vi "Large File - Total Measured Energy.vi"(4 "error in":errorcluster, 7 "tdms file":refnum<k34>) -> (0 "error out":errorcluster, 2 "Total Test Energies (J)":dbl[](array[numeric]), 3 "tdms file out":refnum<k34>)   [LabVIEW 2015]
doc: "Calculates the Total Energy of each shot using Trapezoidal Numeric Integration of the Voltage and Current data. This version deals with the large log files by only reading 100,000 data points from the TDMS file at a time for processing."
uses:
  <vilib>/Analysis/8numeric.llb/1D Numeric Integration.vi
  <vilib>/Analysis/NI_AALPro.lvlib
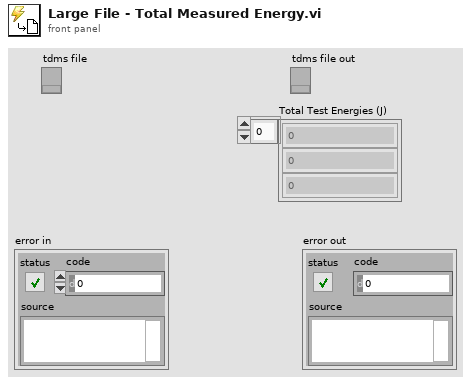
[diagram p1: front panel]
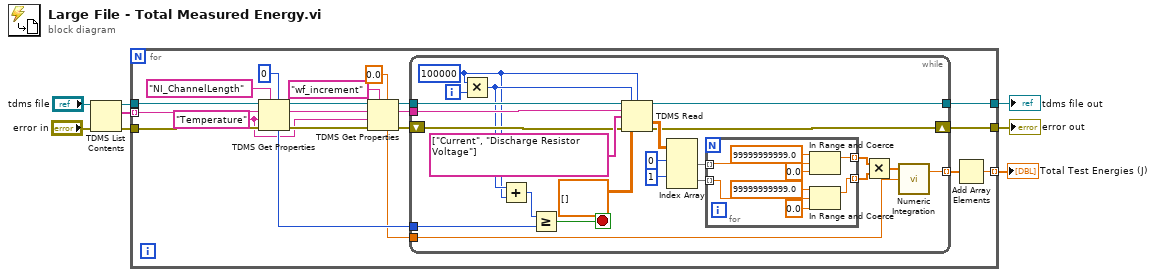
[diagram p0: block diagram]
diagram:
  n1 = TDMS List Contents(4:"error in", 7:"tdms file") -> (0:w7:errorcluster, 2:w6:string[], 3:w8:refnum<k34>)  [unwired: 1 in, 1 out]
  n2 = for {
    tunnel: w8 -> [w22]
    tunnel: [w28] -> w1
    tunnel: w7 -> [w21]
    tunnel: [w27] -> w2
    tunnel: w6 -> [w20] mode=indexing
    tunnel: [w25] -> w5 mode=indexing
    w13 = "Temperature" ("channel name")
    n3 = TDMS Get Properties(5:0, 7:"NI_ChannelLength" ("property name"), 8:w21, 9:w13, 10:w20, 11:w22) -> (0:w18:errorcluster, 2:w16:string, 3:w17:refnum<k34>, 4:w19:i32)  [unwired: 2 out]
    n4 = TDMS Get Properties(5:0.0, 7:"wf_increment" ("property name"), 8:w18, 9:w13, 10:w16, 11:w17) -> (0:w14:errorcluster, 2:w11:string, 3:w15:refnum<k34>, 4:w9:dbl)  [unwired: 2 out]
    n5 = while {
      tunnel: w11 -> [w44]
      tunnel: [w43] -> w26 mode=indexing
      shift-right: [w36] -> w27
      shift-left: w14 -> [w45]
      tunnel: w19 -> [w31]
      tunnel: w15 -> [w46]
      tunnel: [w37] -> w28
      tunnel: w9 -> [w29]
      i -> [w35]
      stop <- w30 stop-if-true
      w33 = i64 100000
      n6 = Multiply(x=w33, y=w35) -> (x*y=w34:i64)
      n7 = Add(x=w34, y=w33) -> (x+y=w32:i64)
      n8 = Greater Or Equal?(x=w32, y=w31) -> (x >= y?=w30:bool)
      n9 = TDMS Read(0:w46, 1:w34, 2:w33, 5:w44, 7:string[] ["Current", "Discharge Resistor Voltage"] ("channel name(s) in"), 11:w45, 12:dbl[][] []) -> (4:w37:refnum<k34>, 10:w42:dbl[][], 15:w36:errorcluster)  [unwired: 1 in, 3 out]
      n10 = Index Array(array=w42, index (row) #1=0 ("index (row)"), index (row) #2=1 ("index (row)")) -> (element #1=w41:dbl[], element #2=w40:dbl[])  [unwired: 2 in]
      n11 = for {
        tunnel: w41 -> [w59] mode=indexing
        tunnel: w40 -> [w56] mode=indexing
        tunnel: [w55] -> w39 mode=indexing
        tunnel: [w54] -> w38 mode=indexing
        n12 = In Range and Coerce(upper limit=99999999999.0, x=w59, lower limit=0.0) -> (coerced(x)=w55:dbl)  [unwired: 1 out]
        n13 = In Range and Coerce(upper limit=99999999999.0, x=w56, lower limit=0.0) -> (coerced(x)=w54:dbl)  [unwired: 1 out]
      }
      n14 = Multiply(x=w39, y=w38) -> (x*y=w51:dbl[])
      n15 = call-poly <vilib>:"Numeric Integration.vi"("dt"=w29, "Input Array"=w51) -> ("result"=w43:dbl)  [unwired: 1 in, 1 out]
    }
    n16 = Add Array Elements(numeric array=w26) -> (sum=w25:dbl)
  }
  "Total Test Energies (J)" <- w5
  "tdms file out" <- w1
  "error out" <- w2
